vi "volumeOpenAndDisplay.vi"() -> ()   [LabVIEW 2017]
uses:
  opencvSegmentConvertCoordinates-multiFrames.vi
  opencvSelectCandidateNeurons5Planes.vi
  opencvSegment.vi
  opencvSegmentConvertCoordinates-singleFrame.vi
  <vilib>/Utility/file.llb/Read Delimited Spreadsheet (I64).vi
  <vilib>/Utility/file.llb/Read Delimited Spreadsheet (DBL).vi
  globalUtilities.vi
panel:
  out "pharosTimes":dbl[](array[numeric])
  in  "transpose":bool
  out "size(s) 3":i32
  out "size(s) 2":i32[](array[numeric])
  in  "times?":bool
  in  "positions?":bool
  out "path":string
  out "size(s)":dbl format="%.2f"
  in  "segment":bool
  in  "#frames":i32
  in  "frame0":i32
  # "RUN THIS VI, SELECT THE FILE\nFROM THE PROMPT AND THEN\nOPEN acquisitionDisplayVolume.vi"
  # "1. frames.dat\n3. pharos trigs\n4. frame details\n2. galvo pos"
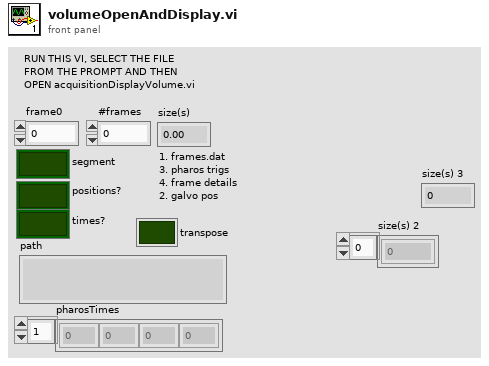
[diagram p1: front panel]
types:
  T1 = enum16{"big-endian, network order", "native, host order", "little-endian"}
  T2 = enum16{"open", "replace", "create", "open or create", "replace or create", "replace or create with confirmation"}
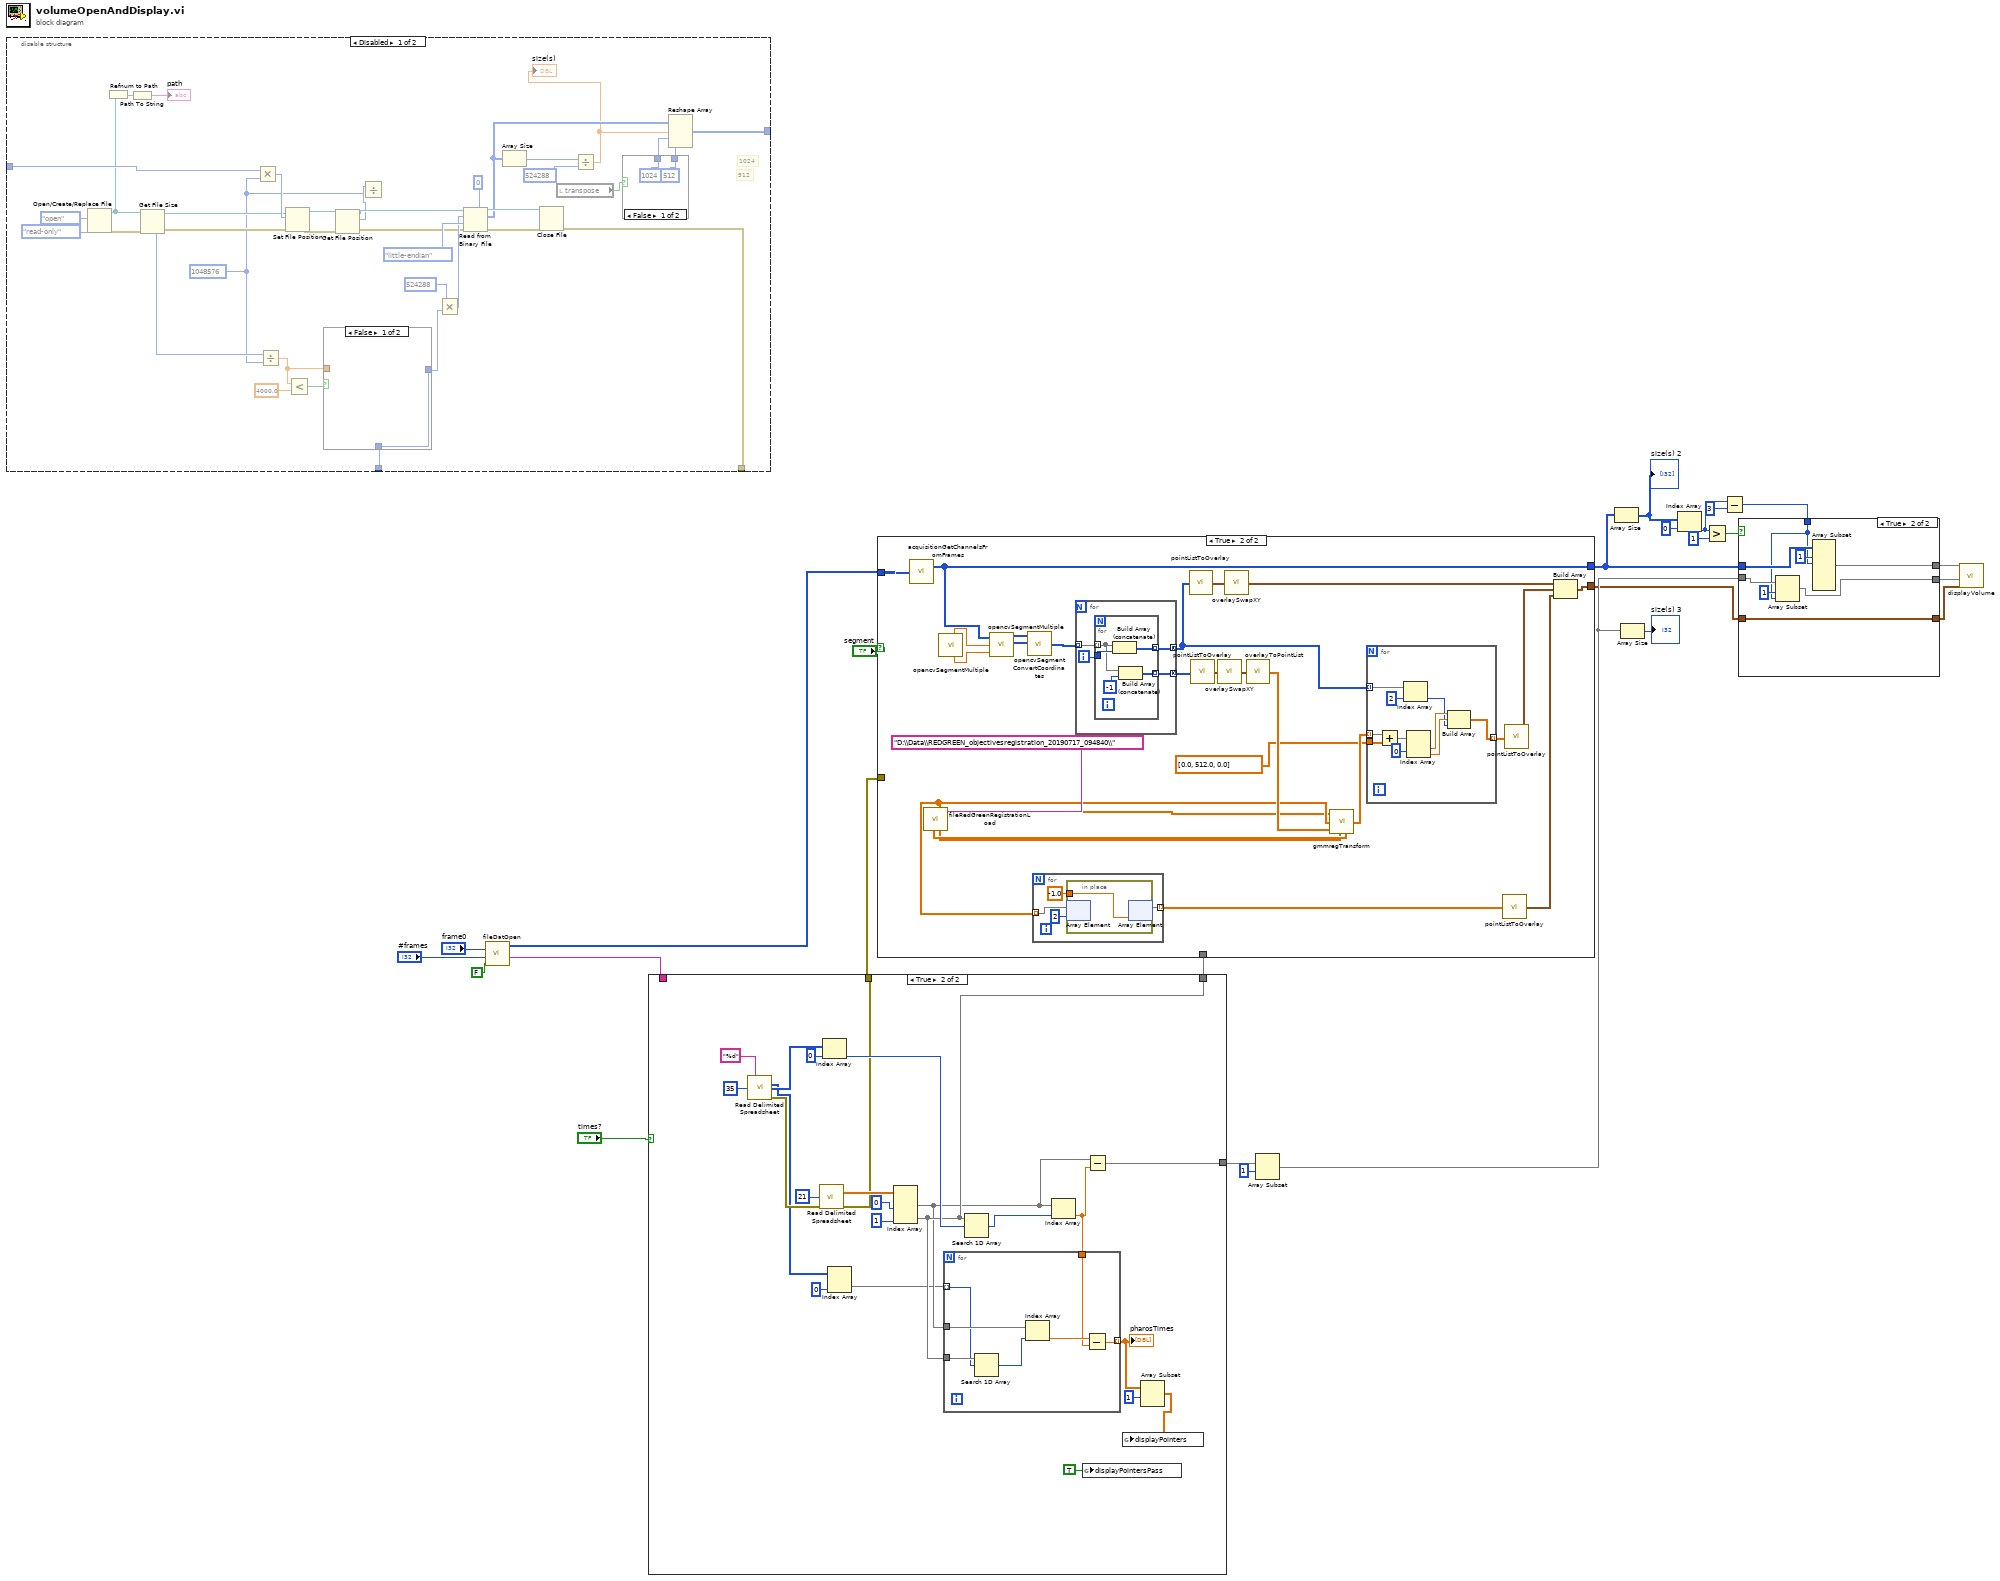
[diagram p0: block diagram]
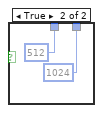
[diagram p2: hidden frame]
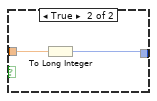
[diagram p3: hidden frame]
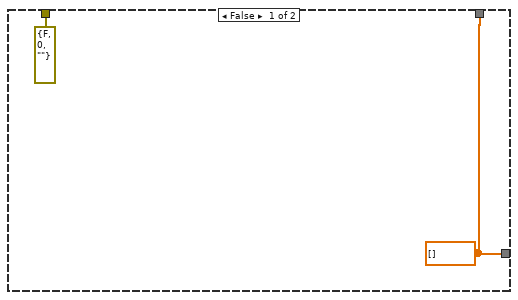
[diagram p6: hidden frame]
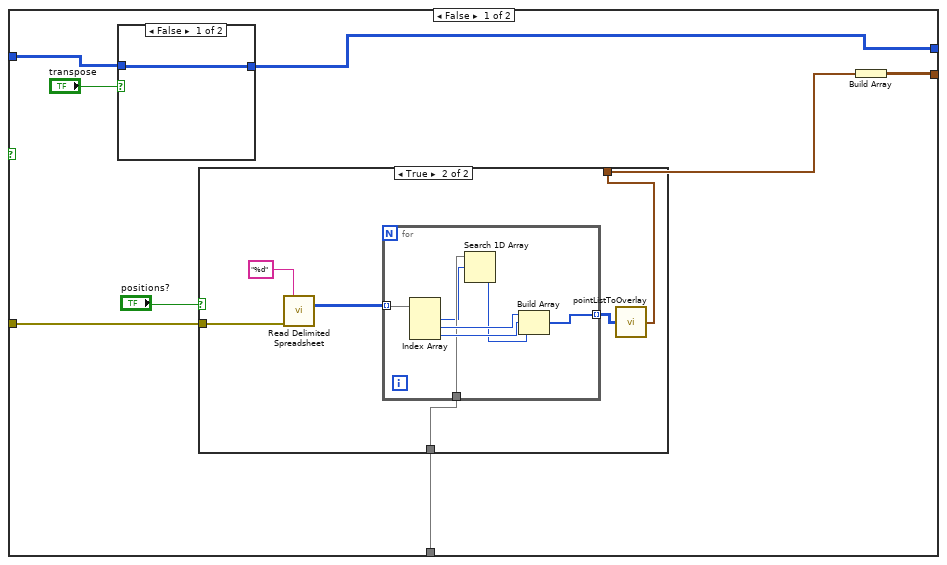
[diagram p7: hidden frame]
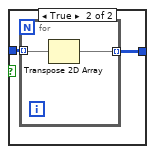
[diagram p8: hidden frame]
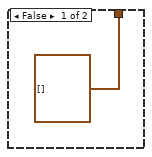
[diagram p9: hidden frame]
diagram:
  n1 = disable-structure shown="Disabled" {
    disable-tunnel: _ -> [w50 _]
    disable-tunnel: [w36 _] -> _
    disable-tunnel: [w29 _] -> _
    disable-tunnel: _ -> [w27 _]
    frame Disabled {
      w37 = 1048576 ("x")
      # "512"
      # "1024"
      n2 = Open/Create/Replace File(operation (0:open)=T2."open", access (0:read/write)=enum16{"read/write", "read-only", "write-only"}."read-only") -> (refnum out=w31:refnum<file>, error out=w48:errorcluster)  [unwired: 4 in, 1 out]
      n3 = Refnum to Path(1:w31) -> (0:w32:path)
      n4 = Path To String(path=w32) -> (string=→"path":string)
      n5 = Get File Size(file=w31, error in=w48) -> (refnum out=w47:refnum<file>, size (in bytes)=w45:i64, 0:w46:errorcluster)
      n6 = Multiply(x=w50, y=w37) -> (x*y=w49:i32)
      n7 = Divide(x=w45, y=w37) -> (x/y=w33:dbl)
      n8 = Set File Position(offset (in bytes) (0)=w49, refnum=w47, error in=w46) -> (refnum out=w42:refnum<file>, error out=w41:errorcluster)  [unwired: 1 in]
      n9 = Less?(x=w33, y=4000.0) -> (x < y?=w34:bool)
      n10 = case shown="False" w34 {
        tunnel: [w67 w68] -> w26
        tunnel: w33 -> [_ w69]
        tunnel: w27 -> [w67 _]
        frame False {
        }
        frame True {
          n11 = To Long Integer(number=w69) -> (32bit integer=w68:i32)
        }
      }
      n12 = Get File Position(4:w41, 7:w42) -> (0:w39:errorcluster, 2:w38:i64, 3:w40:refnum<file>)
      n13 = Divide(x=w38, y=w37) -> ()  [unwired: 1 out]
      n14 = Multiply(x=524288 ("y"), y=w26) -> (x*y=w51:i32)
      n15 = Read from Binary File(5:u16 0, 8:w39, 9:T1."little-endian" ("byte order (0:big-endian, network order)"), 10:w51, 11:w40) -> (0:w57:errorcluster, 2:w56:u16[], 3:w58:refnum<file>)  [unwired: 1 in, 1 out]
      n16 = Array Size(array=w56) -> (size(s)=w55:i32)
      n17 = Close File(refnum=w58, error in=w57) -> (error out=w29:errorcluster)  [unwired: 1 out]
      n18 = local read "transpose"() -> (w28:bool)
      n19 = Divide(x=w55, y=524288) -> (x/y=w44:dbl)
      "size(s)" <- w44
      n20 = case shown="False" w28 {
        tunnel: [1024 ("dimension size") 512 ("dimension size")] -> w53
        tunnel: [512 ("dimension size") 1024 ("dimension size")] -> w52
        frame False {
        }
        frame True {
        }
      }
      n21 = Reshape Array(w56, w44, w53, w52) -> (w36:u16[][][])
    }
    frame Enabled {
    }
  }
  n22 = call "fileDatOpen.vi"("transpose"=FALSE, "#frames"="#frames", "frame0"="frame0") -> ("path"=w2:string, "output array"=w3:u16[][][])  [unwired: 1 in, 2 out]
  n23 = case shown="True" "times?" {
    tunnel: [w71 w84] -> w22
    tunnel: [errorcluster {"status"=FALSE, "code"=0, "source"=""} ("error out") w83] -> w20
    tunnel: [w71 w81] -> w19
    tunnel: w2 -> [_ _]
    frame False {
      w71 = dbl[] []
    }
    frame True {
      n24 = call-poly <vilib>:"Read Delimited Spreadsheet.vi"("format (%d)"="%d" ("format (%.3f)"), "start of read offset (chars.:0)"=35) -> ("all rows"=w78:i64[][], "first row"=w82:i64[], "error out"=w91:errorcluster)  [unwired: 8 in, 3 out]
      n25 = call-poly <vilib>:"Read Delimited Spreadsheet.vi"("start of read offset (chars.:0)"=21, "error in (no error)"=w91) -> ("all rows"=w89:dbl[][], "error out"=w83:errorcluster)  [unwired: 8 in, 4 out]
      n26 = Index Array(array=w82, index=0) -> (element=w88:i64)
      n27 = Index Array(array=w78, index (col)=0 ("disabled index (col)")) -> (element=w76:i64[])  [unwired: 1 in]
      n28 = Index Array(array=w89, index (col) #1=0 ("index (row)"), index (col) #2=1 ("disabled index (col)")) -> (element #1=w80:dbl[], element #2=w81:dbl[])  [unwired: 2 in]
      n29 = Search 1D Array(1D array=w81, element=w88) -> (index of element=w86:i32)  [unwired: 1 in]
      n30 = Index Array(array=w80, index=w86) -> (element=w79:dbl)
      n31 = for {
        tunnel: w76 -> [w95] mode=indexing
        tunnel: w81 -> [w101]
        tunnel: w80 -> [w100]
        tunnel: w79 -> [w97]
        tunnel: [w96] -> w75 mode=indexing
        n32 = Search 1D Array(1D array=w101, element=w95) -> (index of element=w99:i32)  [unwired: 1 in]
        n33 = Index Array(array=w100, index=w99) -> (element=w98:dbl)
        n34 = Subtract(x=w98, y=w97) -> (x-y=w96:dbl)
      }
      "pharosTimes" <- w75
      n35 = global write "globalUtilities.vi" "displayPointersPass"(TRUE ("displayPointersPass")) -> ()
      n36 = Subtract(x=w80, y=w79) -> (x-y=w84:dbl[])
      n37 = Array Subset(array=w75, index=1) -> (w72:dbl[])  [unwired: 1 in]
      n38 = global write "globalUtilities.vi" "displayPointers"(w72) -> ()
    }
  }
  n39 = case shown="True" "segment" {
    tunnel: [w102 w145] -> w1
    tunnel: [w108 w149] -> w18
    tunnel: w3 -> [w109 w148]
    tunnel: w20 -> [w106 _]
    tunnel: w19 -> [w105 _]
    frame False {
      n40 = case shown="False" "transpose" {
        tunnel: w109 -> [w110 w112]
        tunnel: [w110 w111] -> w108
        frame False {
        }
        frame True {
          n41 = for {
            tunnel: w112 -> [w114] mode=indexing
            tunnel: [w113] -> w111 mode=indexing
            n42 = Transpose 2D Array(2D array=w114) -> (transposed array=w113:u16[][])
          }
        }
      }
      n43 = case shown="True" "positions?" {
        tunnel: [cluster{"X":i32, "Y":i32, "Z":i32}[] [] ("overlay (XYZ)") w118] -> w103
        tunnel: w106 -> [_ w117]
        tunnel: w105 -> [_ w116]
        frame False {
        }
        frame True {
          n44 = call-poly <vilib>:"Read Delimited Spreadsheet.vi"("format (%d)"="%d" ("format (%.3f)"), "error in (no error)"=w117) -> ("all rows"=w120:i64[][])  [unwired: 8 in, 5 out]
          n45 = for {
            tunnel: w120 -> [w128] mode=indexing
            tunnel: [w125] -> w119 mode=indexing
            tunnel: w116 -> [w124]
            n46 = Index Array(array=w128) -> (element #1=w123:i64, element #2=w127:i64, element #3=w126:i64)  [unwired: 3 in]
            n47 = Search 1D Array(1D array=w124, element=w123) -> (index of element=w122:i32)  [unwired: 1 in]
            n48 = Build Array(w127, w126, w122) -> (w125:i64[])
          }
          n49 = call "pointListToOverlay.vi"("points"=w119) -> ("overlay (XYZ)"=w118:cluster{"X":i32, "Y":i32, "Z":i32}[])
        }
      }
      n50 = Build Array(w103) -> (w102:cluster{"X":i32, "Y":i32, "Z":i32}[][])
    }
    frame True {
      n51 = call "acquisitionGetChannelsFromFrames.vi"("frameIn"=w148) -> ("Red"=w149:u16[][][])  [unwired: 1 out]
      n52 = call "fileRedGreenRegistrationLoad.vi"("redGreenRegistrationFilePath"="D:\\Data\\REDGREEN_objectivesregistration_20190717_094840\\") -> ("denormParam"=w132:dbl[], "ctrl"=w131:dbl[][], "param"=w130:dbl[], "normParam"=w129:dbl[])  [unwired: 3 in, 2 out]
      n53 = call "opencvSegmentMultiple.vi"() -> ("maxY"=w152:dbl, "maxX"=w151:dbl)  [unwired: 3 in, 4 out]
      n54 = call "opencvSegmentMultiple.vi"("maxYInStack"=w152, "maxXInStack"=w151, "ImgIn"=w149) -> ("NeuronN[frame]"=w154:u16[], "NeuronXY[frame]"=w153:u16[][])  [unwired: 4 out]
      n55 = call-poly "opencvSegmentConvertCoordinates.vi"("NeuronN"=w154, "NeuronXY"=w153) -> ("XY"=w150:u16[][][])  [unwired: 1 in]
      n56 = for {
        tunnel: w131 -> [w168] mode=indexing
        tunnel: [w166] -> w143 mode=indexing
        n57 = in-place {
          in-place-border: -1.0 -> [w169]
          n58 = in-place-array #1(w168, 2) -> ()  [unwired: 1 out]
          n59 = in-place-array #1(w169) -> (w166:dbl[])  [unwired: 1 out]
        }
      }
      n60 = for {
        tunnel: w150 -> [w173] mode=indexing
        tunnel: [w172] -> w134 mode=concatenating
        tunnel: [w170] -> w137 mode=concatenating
        i -> [w171]
        n61 = for {
          tunnel: w173 -> [w176] mode=indexing
          tunnel: [w177] -> w172 mode=indexing
          tunnel: w171 -> [w178]
          tunnel: [w174] -> w170 mode=indexing
          n62 = Build Array (concatenate)(w176, w178) -> (w177:i32[])
          n63 = Build Array (concatenate)(w176, -1) -> (w174:i32[])
        }
      }
      n64 = call "pointListToOverlay.vi"("points"=w134) -> ("overlay (XYZ)"=w147:cluster{"X":i32, "Y":i32, "Z":i32}[])
      n65 = call "pointListToOverlay.vi"("points"=w137) -> ("overlay (XYZ)"=w138:cluster{"X":i32, "Y":i32, "Z":i32}[])
      n66 = call "overlaySwapXY.vi"("overlay in"=w138) -> ("overlay out"=w139:cluster{"X":i32, "Y":i32, "Z":i32}[])
      n67 = call "overlaySwapXY.vi"("overlay in"=w147) -> ("overlay out"=w142:cluster{"X":i32, "Y":i32, "Z":i32}[])
      n68 = call "overlayToPointList.vi"("Overlay"=w139) -> ("PointList"=w136:dbl[][])
      n69 = call "gmmregTransform.vi"("param0"=w130, "ctrlPts"=w131, "pts"=w136, "normParams"=w129, "denormParams"=w132) -> ("out"=w140:dbl[][])  [unwired: 4 in]
      n70 = for {
        tunnel: w140 -> [w164] mode=indexing
        tunnel: [w155] -> w141 mode=indexing
        tunnel: dbl[] [0.0, 512.0, 0.0] -> [w163]
        tunnel: w134 -> [w160] mode=indexing
        n71 = Add(x=w164, y=w163) -> (x+y=w162:dbl[])
        n72 = Index Array(array=w160, index=2) -> (element=w156:i32)
        n73 = Index Array(array=w162, index #1=0 ("index")) -> (element #1=w158:dbl, element #2=w157:dbl)  [unwired: 1 in]
        n74 = Build Array(w158, w157, w156) -> (w155:dbl[])
      }
      n75 = call "pointListToOverlay.vi"("points"=w143) -> ("overlay (XYZ)"=w144:cluster{"X":i32, "Y":i32, "Z":i32}[])
      n76 = call "pointListToOverlay.vi"("points"=w141) -> ("overlay (XYZ)"=w146:cluster{"X":i32, "Y":i32, "Z":i32}[])
      n77 = Build Array(w142, w146, w144) -> (w145:cluster{"X":i32, "Y":i32, "Z":i32}[][])
    }
  }
  n78 = Array Subset(array=w22, index=1) -> (w17:dbl[])  [unwired: 1 in]
  n79 = Array Size(array=w18) -> (size(s)=w16:i32[])
  "size(s) 2" <- w16
  n80 = Array Size(array=w17) -> (size(s)=→"size(s) 3":i32)
  n81 = Index Array(array=w16, index=0) -> (element=w9:i32)
  n82 = Greater?(x=w9, y=1) -> (0:w13:bool)
  n83 = Subtract(x=w9, y=3) -> (x-y=w7:i32)
  n84 = case shown="True" w13 {
    tunnel: w18 -> [w181 w189]
    tunnel: w17 -> [w180 w186]
    tunnel: w1 -> [w179 w183]
    tunnel: [w181 w187] -> w12
    tunnel: [w180 w184] -> w11
    tunnel: [w179 w183] -> w10
    tunnel: w7 -> [_ w182]
    frame False {
    }
    frame True {
      n85 = Array Subset(array=w186, index=1, length=w182) -> (w184:dbl[])
      n86 = Array Subset(array=w189, index (dim 0)=1 ("index"), length (dim 0)=w182) -> (w187:u16[][][])  [unwired: 4 in]
    }
  }
  n87 = call "displayVolume.vi"("frames"=w12, "z"=w11, "overlay (z:-1 all planes)"=w10) -> ()  [unwired: 11 in, 6 out]
